vi "Relative Filepath (File).vi"(6 "SubDirectory?":bool, 8 "error in":errorcluster, 9 "New Directory":string, 10 "Filename":string, 11 "FilePath":path) -> (0 "error out":errorcluster, 2 "Relative FilePath":path)   [LabVIEW 2013]
doc: "Takes a FilePath input, and strips the filename from the path. (If Application strips filename and executable).\nWill then add a new directory if selected and then takes Filename and add to the stripped path."
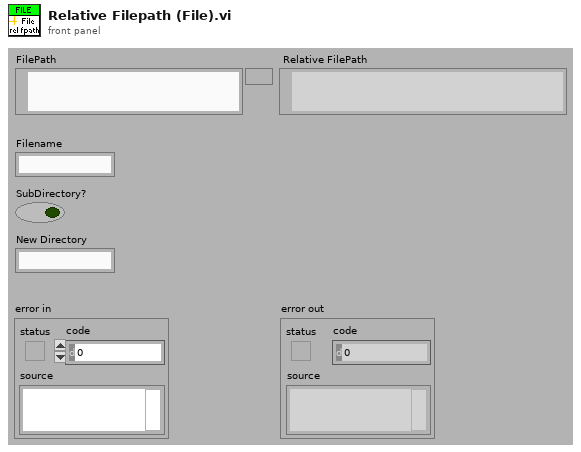
[diagram p1: front panel]
types:
  T1 = enum32{"invalid app kind", "Development System", "Run Time System", "Student Edition", "Embedded LabVIEW", "Evaluation", "Custom"}
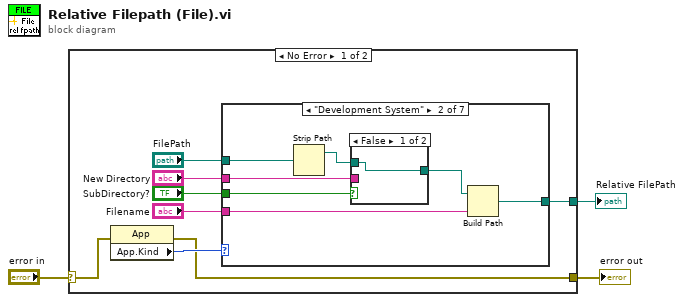
[diagram p0: block diagram]
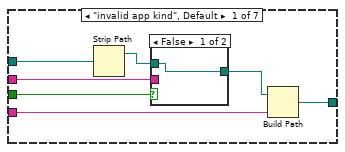
[diagram p2: hidden frame]
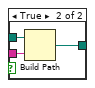
[diagram p3: hidden frame]
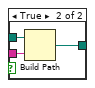
[diagram p4: hidden frame]
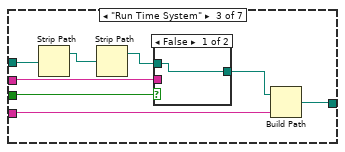
[diagram p5: hidden frame]
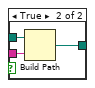
[diagram p6: hidden frame]
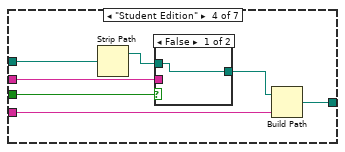
[diagram p7: hidden frame]
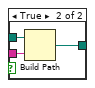
[diagram p8: hidden frame]
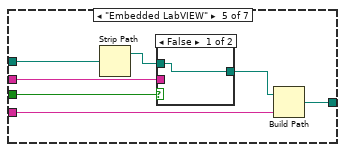
[diagram p9: hidden frame]
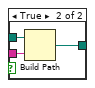
[diagram p10: hidden frame]
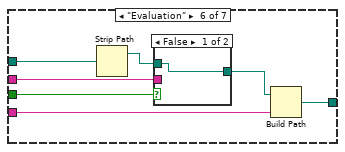
[diagram p11: hidden frame]
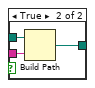
[diagram p12: hidden frame]
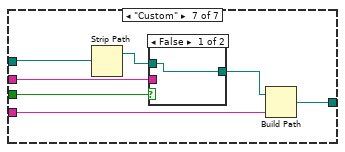
[diagram p13: hidden frame]
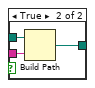
[diagram p14: hidden frame]
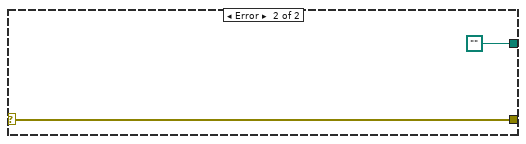
[diagram p15: hidden frame]
diagram:
  n1 = case shown="No Error" "error in" {
    selector: "error in" -> [w6 w91]
    tunnel: [w7 path ""] -> w3
    tunnel: [w5 w91] -> w2
    frame No Error {
      n2 = property class="App"(error in=w6) -> (error out=w5:errorcluster, "App.Kind"=w11:T1)  [unwired: 1 in, 1 out]
      n3 = case shown="\"Development System\"" w11 {
        tunnel: "FilePath" -> [w13 w29 w35 w47 w58 w72 w80]
        tunnel: "New Directory" -> [w16 w27 w39 w50 w61 w71 w83]
        tunnel: "Filename" -> [w14 w25 w37 w48 w59 w69 w81]
        tunnel: [w12 w24 w36 w46 w57 w68 w79] -> w7
        tunnel: "SubDirectory?" -> [w15 w23 w38 w49 w60 w70 w82]
        frame "invalid app kind", Default {
          n4 = Strip Path(path=w13) -> (stripped path=w17:path)  [unwired: 1 out]
          n5 = case shown="False" w15 {
            tunnel: w17 -> [w19 w22]
            tunnel: w16 -> [_ w21]
            tunnel: [w19 w20] -> w18
            frame False {
            }
            frame True {
              n6 = Build Path(base path=w22, name or relative path=w21) -> (appended path=w20:path)
            }
          }
          n7 = Build Path(base path=w18, name or relative path=w14) -> (appended path=w12:path)
        }
        frame "Development System" {
          n8 = Strip Path(path=w29) -> (stripped path=w28:path)  [unwired: 1 out]
          n9 = case shown="False" w23 {
            tunnel: w28 -> [w30 w33]
            tunnel: w27 -> [_ w32]
            tunnel: [w30 w31] -> w26
            frame False {
            }
            frame True {
              n10 = Build Path(base path=w33, name or relative path=w32) -> (appended path=w31:path)
            }
          }
          n11 = Build Path(base path=w26, name or relative path=w25) -> (appended path=w24:path)
        }
        frame "Run Time System" {
          n12 = Strip Path(path=w35) -> (stripped path=w34:path)  [unwired: 1 out]
          n13 = Strip Path(path=w34) -> (stripped path=w41:path)  [unwired: 1 out]
          n14 = case shown="False" w38 {
            tunnel: w41 -> [w42 w45]
            tunnel: w39 -> [_ w44]
            tunnel: [w42 w43] -> w40
            frame False {
            }
            frame True {
              n15 = Build Path(base path=w45, name or relative path=w44) -> (appended path=w43:path)
            }
          }
          n16 = Build Path(base path=w40, name or relative path=w37) -> (appended path=w36:path)
        }
        frame "Student Edition" {
          n17 = Strip Path(path=w47) -> (stripped path=w52:path)  [unwired: 1 out]
          n18 = case shown="False" w49 {
            tunnel: w52 -> [w53 w56]
            tunnel: w50 -> [_ w55]
            tunnel: [w53 w54] -> w51
            frame False {
            }
            frame True {
              n19 = Build Path(base path=w56, name or relative path=w55) -> (appended path=w54:path)
            }
          }
          n20 = Build Path(base path=w51, name or relative path=w48) -> (appended path=w46:path)
        }
        frame "Embedded LabVIEW" {
          n21 = Strip Path(path=w58) -> (stripped path=w63:path)  [unwired: 1 out]
          n22 = case shown="False" w60 {
            tunnel: w63 -> [w64 w67]
            tunnel: w61 -> [_ w66]
            tunnel: [w64 w65] -> w62
            frame False {
            }
            frame True {
              n23 = Build Path(base path=w67, name or relative path=w66) -> (appended path=w65:path)
            }
          }
          n24 = Build Path(base path=w62, name or relative path=w59) -> (appended path=w57:path)
        }
        frame "Evaluation" {
          n25 = Strip Path(path=w72) -> (stripped path=w74:path)  [unwired: 1 out]
          n26 = case shown="False" w70 {
            tunnel: w74 -> [w75 w78]
            tunnel: w71 -> [_ w77]
            tunnel: [w75 w76] -> w73
            frame False {
            }
            frame True {
              n27 = Build Path(base path=w78, name or relative path=w77) -> (appended path=w76:path)
            }
          }
          n28 = Build Path(base path=w73, name or relative path=w69) -> (appended path=w68:path)
        }
        frame "Custom" {
          n29 = Strip Path(path=w80) -> (stripped path=w85:path)  [unwired: 1 out]
          n30 = case shown="False" w82 {
            tunnel: w85 -> [w86 w89]
            tunnel: w83 -> [_ w88]
            tunnel: [w86 w87] -> w84
            frame False {
            }
            frame True {
              n31 = Build Path(base path=w89, name or relative path=w88) -> (appended path=w87:path)
            }
          }
          n32 = Build Path(base path=w84, name or relative path=w81) -> (appended path=w79:path)
        }
      }
    }
    frame Error {
    }
  }
  "Relative FilePath" <- w3
  "error out" <- w2
